vi "Find Start and Endpoint Body Text.vi"(11 "Icon":picture) -> (1 "Pos offset":i32, 2 "Neg offset":i32, 3 "Found?":bool, 5 "Transparent?":bool)   [LabVIEW 2017, in "lv_icon.lvlib"]
doc: "Find the actual start and endpoint of the text to be able to center the Text later on."
uses:
  <vilib>/LabVIEW Icon API/lv_icon/lv_icon.lvlib
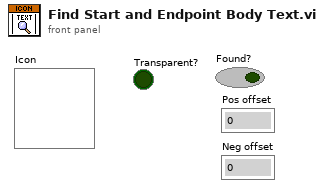
[diagram p1: front panel]
types:
  T1 = cluster{"left":i16, "top":i16, "right":i16, "bottom":i16}
  T2 = typedef "imagedata.ctl" = cluster{"image type":i32, "image depth":i32, "image":u8[], "mask":u8[], "colors":u32[], "Rectangle":cluster{"left":i16, "top":i16, "right":i16, "bottom":i16}}
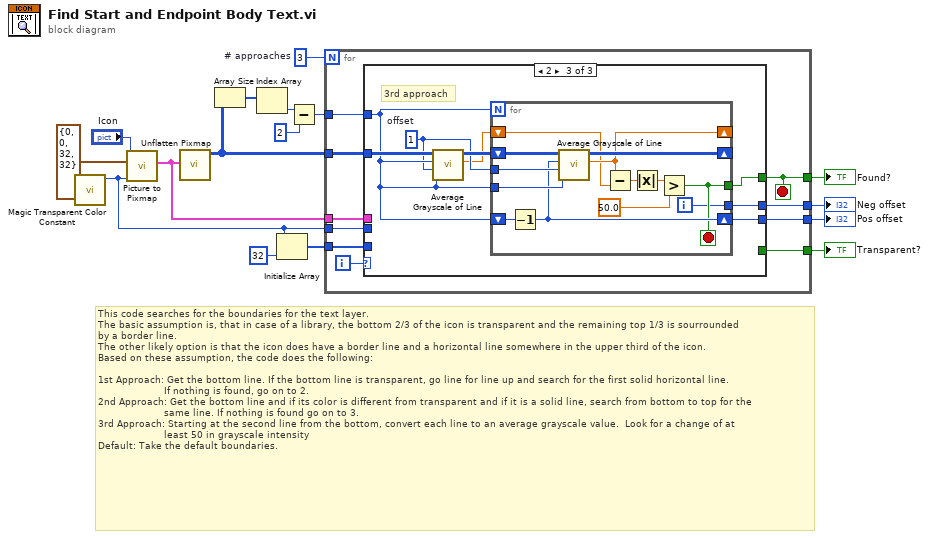
[diagram p0: block diagram]
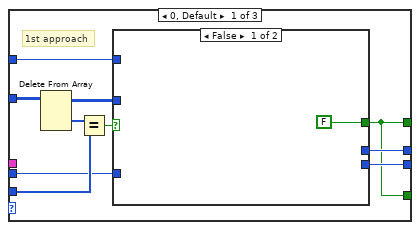
[diagram p2: hidden frame]
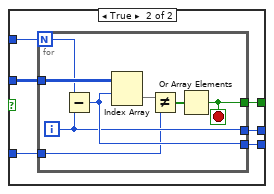
[diagram p3: hidden frame]
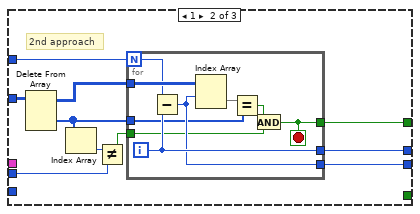
[diagram p4: hidden frame]
diagram:
  w14 = 3  # # approaches
  # "This code searches for the boundaries for the text layer.\nThe basic assumption is, that in case of a library, the bottom 2/3 of the icon is transparent and the remaining top 1/3 is sourrounded\nby a border line.\nThe other likely option is that the icon does have a border line and a horizontal line somewhere in the upper third of the icon.\nBased on these assumption, the code does the following:\n\n1st Approach: Get the bottom line. If the bottom line is transparent, go line for line up and search for the first solid horizontal line.\n                      If nothing is found, go on to 2.\n2nd Approach: Get the bottom line and if its color is different from transparent and if it is a solid line, search from bottom to top for the\n                      same line. If nothing is found go on to 3. \n3rd Approach: Starting at the second line from the bottom, convert each line to an average grayscale value.  Look for a change of at\n                      least 50 in grayscale intensity\nDefault: Take the default boundaries."
  n1 = call <vilib>:"Magic Transparent Color Constant.vi"() -> ("Magic transparent color constant"=w2:u32)  [unwired: 11 out]
  n2 = call <vilib>:"Picture to Pixmap.vi"("Background Color"=w2, "rect"=T1 {"left"=0, "top"=0, "right"=32, "bottom"=32}, "picture"="Icon") -> ("image data"=w6:T2)  [unwired: 1 in, 7 out]
  n3 = call <vilib>:"Unflatten Pixmap.vi"("image data"=w6) -> ("24-bit pixmap"=w13:u32[][])  [unwired: 10 out]
  n4 = Array Size(array=w13) -> (size(s)=w12:i32[])
  n5 = Index Array(array=w12) -> (element=w11:i32)  [unwired: 1 in]
  n6 = Initialize Array(w2, 32 ("dimension size")) -> (w3:u32[])
  n7 = Subtract(x=w11, y=2) -> (x-y=w9:i32)
  n8 = for {
    N: w14 -> [_]
    tunnel: [w26] -> w7
    tunnel: [w22] -> w16
    tunnel: w9 -> [w25]
    tunnel: [w24] -> w8
    tunnel: w13 -> [w23]
    tunnel: w6 -> [w21]
    tunnel: w3 -> [w19]
    tunnel: w2 -> [w18]
    tunnel: [w17] -> w1
    i -> [w20]
    stop <- w22 stop-if-true
    n9 = case shown="2" w20 {
      tunnel: [w33 w61 w78] -> w26
      tunnel: [w27 w60 w72] -> w22
      tunnel: w25 -> [w35 w59 w75]
      tunnel: [w34 w58 w71] -> w24
      tunnel: w23 -> [w36 w56 w76]
      tunnel: w21 -> [_ _ _]
      tunnel: w19 -> [w32 _ _]
      tunnel: w18 -> [w31 w53 _]
      tunnel: [w27 _ _] -> w17
      frame 0, Default {
        # "1st approach"
        n10 = Delete From Array(array=w36) -> (deleted portion=w30:u32[], array with subset deleted=w28:u32[][])  [unwired: 3 in]
        n11 = Equal?(x=w30, y=w32) -> (x = y?=w29:bool)
        n12 = case shown="False" w29 {
          tunnel: w28 -> [_ w42]
          tunnel: w35 -> [_ w43]
          tunnel: [FALSE w41] -> w27
          tunnel: [_ w40] -> w34
          tunnel: [_ w39] -> w33
          tunnel: w31 -> [_ w38]
          frame False {
          }
          frame True {
            n13 = for {
              N: w43 -> [w49]
              tunnel: w42 -> [w51]
              tunnel: [w46] -> w41
              tunnel: [w48] -> w40
              tunnel: [w50] -> w39
              tunnel: w38 -> [w44]
              i -> [w48]
              stop <- w46 stop-if-true
              n14 = Subtract(x=w49, y=w48) -> (x-y=w50:i32)
              n15 = Index Array(array=w51, index (row)=w50) -> (element=w47:u32[])  [unwired: 1 in]
              n16 = Not Equal?(x=w47, y=w44) -> (x != y?=w45:bool[])
              n17 = Or Array Elements(Boolean array=w45) -> (logical OR=w46:bool)
            }
          }
        }
      }
      frame 1 {
        # "2nd approach"
        n18 = Delete From Array(array=w56) -> (deleted portion=w54:u32[], array with subset deleted=w57:u32[][])  [unwired: 3 in]
        n19 = Index Array(array=w54) -> (element=w55:u32)  [unwired: 1 in]
        n20 = Not Equal?(x=w55, y=w53) -> (x != y?=w52:bool)
        n21 = for {
          N: w59 -> [w66]
          tunnel: w57 -> [w70]
          tunnel: w54 -> [w63]
          tunnel: [w64] -> w60
          tunnel: [w69] -> w58
          tunnel: [w67] -> w61
          tunnel: w52 -> [w62]
          i -> [w69]
          stop <- w64 stop-if-true
          n22 = Subtract(x=w66, y=w69) -> (x-y=w67:i32)
          n23 = Index Array(array=w70, index (row)=w67) -> (element=w68:u32[])  [unwired: 1 in]
          n24 = Equal?(x=w68, y=w63) -> (x = y?=w65:bool)
          n25 = And(x=w65, y=w62) -> (x .and. y?=w64:bool)
        }
      }
      frame 2 {
        w74 = 1  # offset
        # "3rd approach"
        n26 = call <vilib>:"Average Grayscale of Line.vi"("nPoints"=w75, "offset"=w74, "row"=w75, "24-bit pixmap in"=w76) -> ("average grayscale"=w73:sgl, "24-bit pixmap out"=w77:u32[][])  [unwired: 6 in]
        n27 = for {
          N: w75 -> [_]
          shift-right: [w86] -> _
          shift-left: w77 -> [w91]
          shift-right: [w87] -> w78
          shift-left: w75 -> [w90]
          tunnel: w75 -> [w88]
          tunnel: w74 -> [w89]
          shift-right: [w85] -> _
          shift-left: w73 -> [w84]
          tunnel: [w80] -> w72
          tunnel: [w79] -> w71
          i -> [w79]
          stop <- w80 stop-if-true
          n28 = Decrement(x=w90) -> (x-1=w87:i32)
          n29 = call <vilib>:"Average Grayscale of Line.vi"("nPoints"=w88, "offset"=w89, "row"=w87, "24-bit pixmap in"=w91) -> ("average grayscale"=w85:sgl, "24-bit pixmap out"=w86:u32[][])  [unwired: 6 in]
          n30 = Subtract(x=w85, y=w84) -> (x-y=w83:sgl)
          n31 = Absolute Value(x=w83) -> (abs(x)=w82:sgl)
          n32 = Greater?(x=w82, y=sgl 50.0) -> (0:w80:bool)
        }
      }
    }
  }
  "Pos offset" <- w7
  "Found?" <- w16
  "Neg offset" <- w8
  "Transparent?" <- w1
